vi "driver test.vi"() -> ()   [LabVIEW 2016]
panel:
  out "Send Position":dbl[](array[numeric])
  in  "stop":bool
  out "Curent Position":dbl[](array[numeric])
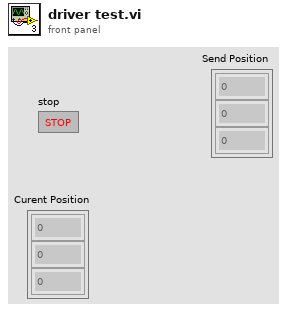
[diagram p1: front panel]
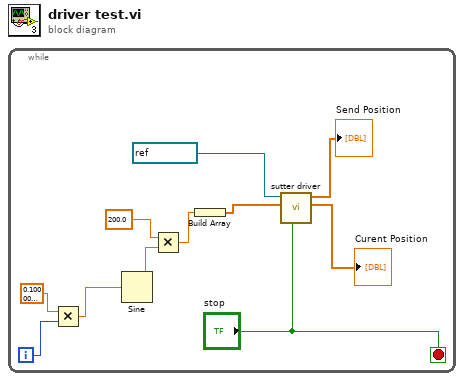
[diagram p0: block diagram]
diagram:
  n1 = while {
    i -> [w9]
    stop <- "stop" stop-if-true
    n2 = Multiply(x=sgl 0.1, y=w9) -> (x*y=w7:sgl)
    n3 = Sine(x=w7) -> (sin(x)=w6:sgl)
    n4 = Multiply(x=sgl 200.0, y=w6) -> (x*y=w4:sgl)
    n5 = Build Array(w4) -> (w3:sgl[])
    n6 = call "sutter driver.vi"("stop"="stop", "Pos error"=w3, "VISA resource name"=refnum<visa-resource-name> "COM1") -> ("Curent Position"=→"Curent Position":dbl[], "Send Position"=→"Send Position":dbl[])  [unwired: 3 in, 1 out]
  }
